vi "DetectorP2.vi"() -> ()   [LabVIEW 2018]
panel:
  in  "Number of Trajectories (x3)":i64
  in  "Number of Pixels":i64
  out "Intensity Graph 2":dbl[][](graph)
  out "XY Graph":cluster{dbl[], dbl[]}(graph)
  in  "height":dbl
  in  "eField":dbl
  in  "bField":dbl
  in  "velocity":dbl
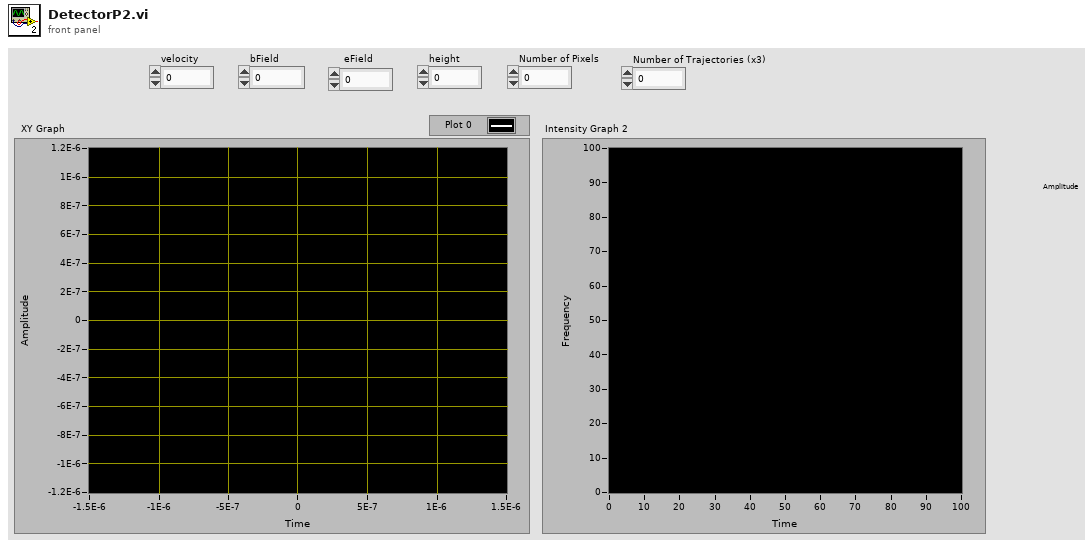
[diagram p1: front panel]
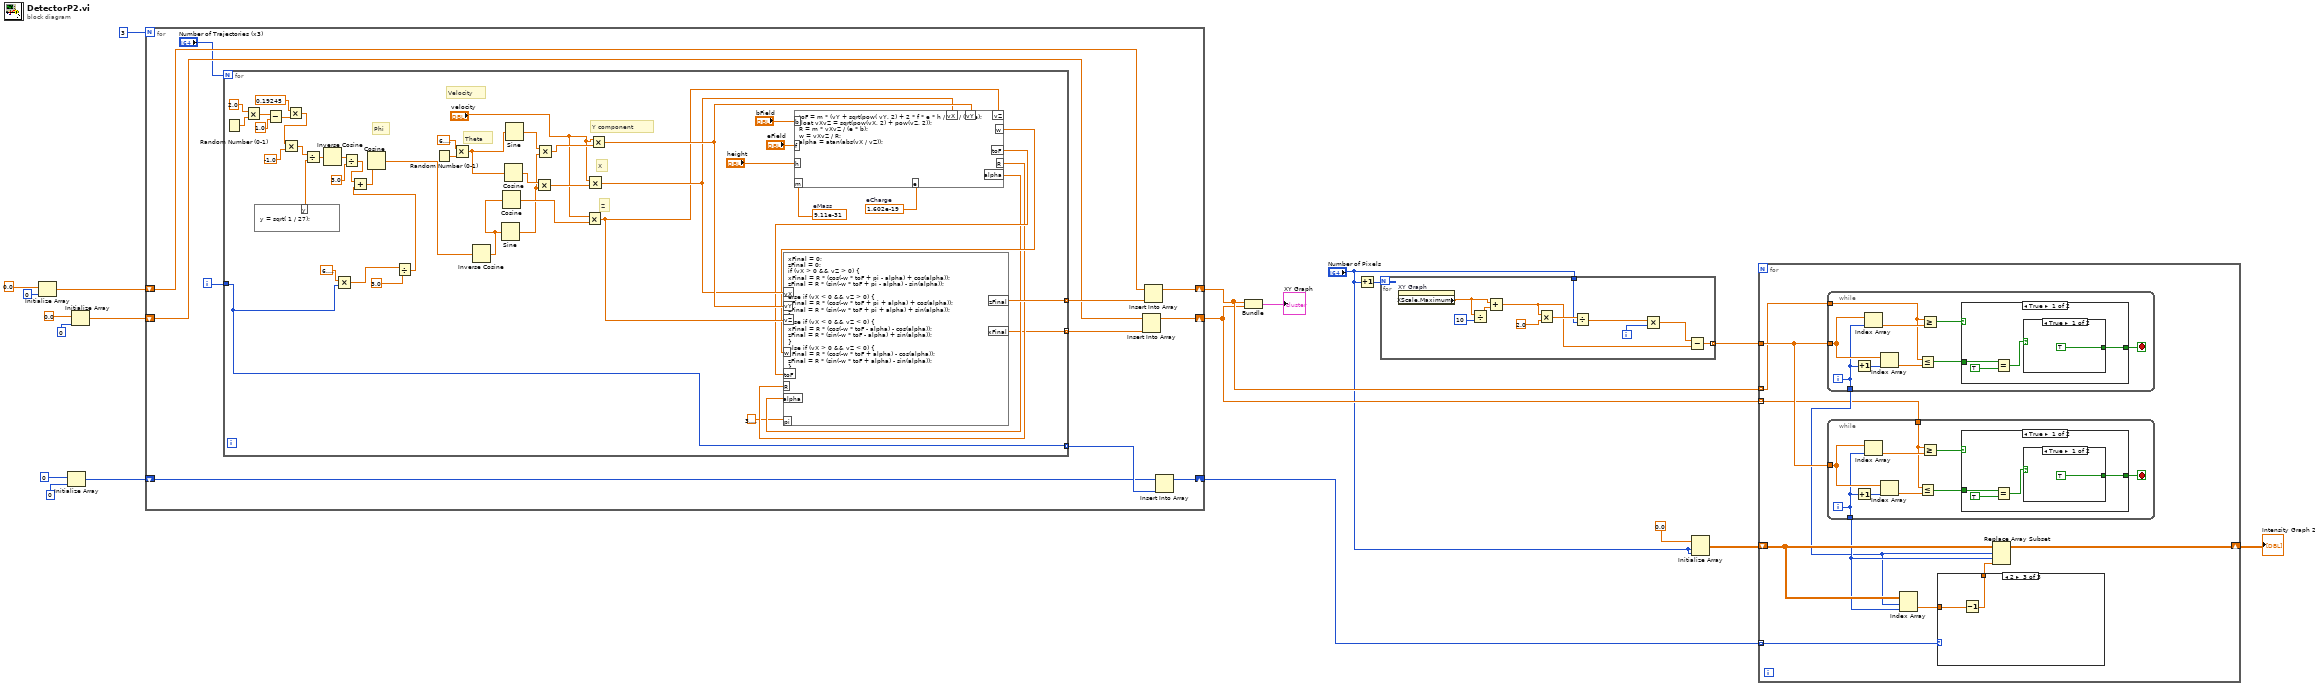
[diagram p0: block diagram]
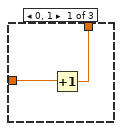
[diagram p2: hidden frame]
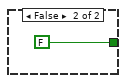
[diagram p4: hidden frame]
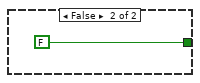
[diagram p5: hidden frame]
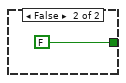
[diagram p6: hidden frame]
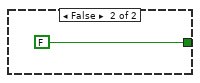
[diagram p7: hidden frame]
diagram:
  n1 = Initialize Array(0.0, 0) -> (w15:dbl[])
  n2 = Initialize Array(0, 0) -> (w11:i32[])
  n3 = Initialize Array(0.0, 0) -> (w14:dbl[])
  n4 = for {
    N: 3 -> [_]
    shift-right: [w30] -> w3
    shift-left: w15 -> [w26]
    shift-right: [w29] -> w2
    shift-left: w14 -> [w25]
    shift-right: [w22] -> w4
    shift-left: w11 -> [w23]
    i -> [w31]
    n5 = for {
      N: "Number of Trajectories (x3)" -> [_]
      tunnel: w31 -> [w32]
      tunnel: [w44] -> w27 mode=indexing
      tunnel: [w33] -> w28 mode=indexing
      tunnel: [w32] -> w24 mode=indexing
      w34 = 1.602e-19  # eCharge
      w39 = 9.11e-31  # eMass
      # "Phi"
      # "Theta"
      # "Z"
      # "X"
      # "Y component"
      # "Velocity"
      n6 = Random Number (0-1)() -> (number: 0 to 1=w58:dbl)
      n7 = Multiply(x=2.0, y=w58) -> (x*y=w59:dbl)
      n8 = formula code="y = sqrt( 1 / 27);"() -> ("y"=w50:dbl)
      n9 = Subtract(x=w59, y=1.0) -> (x-y=w60:dbl)
      n10 = Multiply(x=0.19245, y=w60) -> (x*y=w61:dbl)
      n11 = Multiply(x=w61, y=-1.0) -> (x*y=w57:dbl)
      n12 = Divide(x=w57, y=w50) -> (x/y=w63:dbl)
      n13 = Inverse Cosine(1:w63) -> (0:w62:dbl)
      n14 = Multiply(x=6.283185307179586, y=w32) -> (x*y=w48:dbl)
      n15 = Divide(x=w62, y=3.0) -> (x/y=w64:dbl)
      n16 = Divide(x=w48, y=3.0) -> (x/y=w46:dbl)
      n17 = Add(x=w64, y=w46) -> (x+y=w65:dbl)
      n18 = Cosine(x=w65) -> (cos(x)=w51:dbl)
      n19 = Random Number (0-1)() -> (number: 0 to 1=w78:dbl)
      n20 = Multiply(x=6.283185307179586, y=w78) -> (x*y=w76:dbl)
      n21 = Inverse Cosine(1:w51) -> (0:w67:dbl)
      n22 = Sine(x=w67) -> (sin(x)=w69:dbl)
      n23 = Cosine(x=w67) -> (cos(x)=w73:dbl)
      n24 = Cosine(x=w76) -> (cos(x)=w70:dbl)
      n25 = Sine(x=w76) -> (sin(x)=w72:dbl)
      n26 = Multiply(x=w70, y=w69) -> (x*y=w68:dbl)
      n27 = Multiply(x=w72, y=w69) -> (x*y=w71:dbl)
      n28 = Multiply(x="velocity", y=w73) -> (x*y=w66:dbl)
      n29 = Multiply(x="velocity", y=w68) -> (x*y=w74:dbl)
      n30 = Multiply(x="velocity", y=w71) -> (x*y=w75:dbl)
      n31 = formula code="toF = m * (vY + sqrt(pow( vY, 2) + 2 * f * e * h / m)) / (f * e);\nfloat vXvZ = sqrt(pow(vX, 2) + pow(vZ, 2));\nR = m * vXvZ / (e * b);\nw = vXvZ / R;\nalpha = atan(abs(vX / vZ));"("f"="eField", "h"="height", "vY"=w75, "m"=w39, "e"=w34, "vX"=w74, "vZ"=w66, "b"="bField") -> ("toF"=w43:dbl, "w"=w42:dbl, "R"=w41:dbl, "alpha"=w40:dbl)
      n32 = formula code="xFinal = 0;\nzFinal = 0;\nif (vX > 0 && vZ > 0) {\nxFinal = R * (cos(-w * toF + pi - alpha) + cos(alpha));\nzFinal = R * (sin(-w * toF + pi - alpha) - sin(alpha));\n}\nelse if (vX < 0 && vZ > 0) {\nxFinal = R * (cos(-w * toF + pi + alpha) + cos(alpha));\nzFinal = R * (sin(-w * toF + pi + alpha) + sin(alpha));\n}\nelse if (vX < 0 && vZ < 0) {\nxFinal = R * (cos(-w * toF - alpha) - cos(alpha));\nzFinal = R * (sin(-w * toF - alpha) + sin(alpha));\n}\nelse if (vX > 0 && vZ < 0) {\nxFinal = R * (cos(-w * toF + alpha) - cos(alpha));\nzFinal = R * (sin(-w * toF + alpha) - sin(alpha));\n}"("vY"=w75, "toF"=w43, "vX"=w74, "vZ"=w66, "w"=w42, "R"=w41, "alpha"=w40, "pi"=3.141592653589793) -> ("zFinal"=w44:dbl, "xFinal"=w33:dbl)
    }
    n33 = Insert Into Array(array=w25, new element=w28) -> (w29:dbl[])  [unwired: 1 in]
    n34 = Insert Into Array(array=w26, new element=w27) -> (w30:dbl[])  [unwired: 1 in]
    n35 = Insert Into Array(array=w23, new element=w24) -> (w22:i32[])  [unwired: 1 in]
  }
  n36 = Bundle(w3, w2) -> (→"XY Graph":cluster{dbl[], dbl[]})  [unwired: 1 in]
  n37 = Increment(x="Number of Pixels") -> (x+1=w9:i64)
  n38 = for {
    N: w9 -> [_]
    tunnel: [w89] -> w8 mode=indexing
    tunnel: "Number of Pixels" -> [w86]
    i -> [w85]
    n39 = property on="XY Graph" class="XYGraph (strict)"() -> ("XScale.Maximum"=w79:dbl)  [unwired: 2 in, 2 out]
    n40 = Divide(x=w79, y=10) -> (x/y=w81:dbl)
    n41 = Add(x=w79, y=w81) -> (x+y=w80:dbl)
    n42 = Multiply(x=w80, y=2.0) -> (x*y=w87:dbl)
    n43 = Divide(x=w87, y=w86) -> (x/y=w84:dbl)
    n44 = Multiply(x=w84, y=w85) -> (x*y=w83:dbl)
    n45 = Subtract(x=w83, y=w80) -> (x-y=w89:dbl)
  }
  n46 = Initialize Array(0.0, "Number of Pixels", "Number of Pixels") -> (w7:dbl[][])
  n47 = for {
    tunnel: w8 -> [w99]
    shift-right: [w93] -> w5
    shift-left: w7 -> [w96]
    tunnel: w4 -> [w92] mode=indexing
    tunnel: w3 -> [w91] mode=indexing
    tunnel: w2 -> [w90] mode=indexing
    n48 = while {
      tunnel: w99 -> [w129]
      tunnel: [w124] -> w94
      tunnel: w91 -> [w121]
      i -> [w124]
      stop <- w123 stop-if-true
      n49 = Increment(x=w124) -> (x+1=w128:i32)
      n50 = Index Array(array=w129, index=w124) -> (element=w127:dbl)
      n51 = Index Array(array=w129, index=w128) -> (element=w126:dbl)
      n52 = Less Or Equal?(x=w121, y=w126) -> (x <= y?=w125:bool)
      n53 = Greater Or Equal?(x=w121, y=w127) -> (x >= y?=w122:bool)
      n54 = case shown="True" w122 {
        tunnel: w125 -> [w132 _]
        tunnel: [w130 FALSE] -> w123
        frame True {
          n55 = Equal?(x=w132, y=TRUE) -> (x = y?=w131:bool)
          n56 = case shown="True" w131 {
            tunnel: [TRUE FALSE] -> w130
            frame True {
            }
            frame False {
            }
          }
        }
        frame False {
        }
      }
    }
    n57 = while {
      tunnel: w99 -> [w113]
      tunnel: [w108] -> w95
      tunnel: w90 -> [w105]
      i -> [w108]
      stop <- w107 stop-if-true
      n58 = Increment(x=w108) -> (x+1=w112:i32)
      n59 = Index Array(array=w113, index=w108) -> (element=w111:dbl)
      n60 = Index Array(array=w113, index=w112) -> (element=w110:dbl)
      n61 = Less Or Equal?(x=w105, y=w110) -> (x <= y?=w109:bool)
      n62 = Greater Or Equal?(x=w105, y=w111) -> (x >= y?=w106:bool)
      n63 = case shown="True" w106 {
        tunnel: w109 -> [w116 _]
        tunnel: [w114 FALSE] -> w107
        frame True {
          n64 = Equal?(x=w116, y=TRUE) -> (x = y?=w115:bool)
          n65 = case shown="True" w115 {
            tunnel: [TRUE FALSE] -> w114
            frame True {
            }
            frame False {
            }
          }
        }
        frame False {
        }
      }
    }
    n66 = Index Array(array=w96, index (row)=w94, index (col)=w95) -> (element=w97:dbl)
    n67 = case shown="2" w92 {
      tunnel: [w101 w102 w104] -> w98
      tunnel: w97 -> [w100 w102 w103]
      frame 0, 1 {
        n68 = Increment(x=w100) -> (x+1=w101:dbl)
      }
      frame Default {
      }
      frame 2 {
        n69 = Decrement(x=w103) -> (x-1=w104:dbl)
      }
    }
    n70 = Replace Array Subset(array=w96, new element=w98, index (row)=w94, index (col)=w95) -> (w93:dbl[][])
  }
  "Intensity Graph 2" <- w5
